vi "zmq_config_curve.vi"(4 "domain (none)":string, 5 "server public":string, 6 "error in":errorcluster, 7 "public in":string, 8 "secret in":string, 9 "socket in":refnum<class "Socket.lvclass">) -> (0 "error out":errorcluster, 1 "public out":string, 2 "secret out":string, 3 "socket out":refnum<class "Socket.lvclass">)   [LabVIEW 2025, in "ZeroMQ.lvlib" / "Socket.lvclass"]
doc: "Configures a socket for CURVE authentication. If the server (public) key is provided, then the socket is configured as a client, otherwise it is configured as a server.\n\nPublic and private keys can be manually specified, and are automatically generated if not provided.\n\nKeys are encoded in Z85 format.\n\nDomain <b>should</b> be specified for authentication purposes.\n\nDetailed API documentation: http://api.zeromq.org/master:zmq-curve"
uses:
  Socket.lvclass
  Socket.lvclass/Socket.ctl
  socket_options.ctl
  ZeroMQ.lvlib
panel:
  # "ØMQ"
  # "labview"
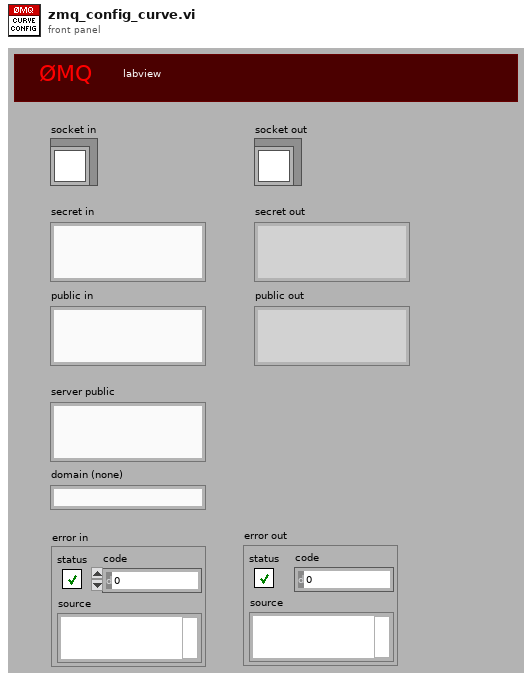
[diagram p1: front panel]
types:
  T1 = typedef "ZeroMQ.lvlib/socket_options.ctl" = enum8{"NONE", "ZMQ_HWM", "<2>", "ZMQ_SWAP", "ZMQ_AFFINITY", "ZMQ_ROUTING_ID", "ZMQ_SUBSCRIBE", "ZMQ_UNSUBSCRIBE", "ZMQ_RATE", "ZMQ_RECOVERY_IVL", "ZMQ_MCAST_LOOP", "ZMQ_SNDBUF", "ZMQ_RCVBUF", "ZMQ_RCVMORE", "ZMQ_FD", "ZMQ_EVENTS", "ZMQ_TYPE", "ZMQ_LINGER", "ZMQ_RECONNECT_IVL", "ZMQ_BACKLOG", "ZMQ_RECOVERY_IVL_MSEC", "ZMQ_RECONNECT_IVL_MAX", "ZMQ_MAXMSGSIZE", "ZMQ_SNDHWM", "ZMQ_RCVHWM", "ZMQ_MULTICAST_HOPS", "<26>", "ZMQ_RCVTIMEO", "ZMQ_SNDTIMEO", "<29>", "<30>", "ZMQ_IPV4ONLY", "ZMQ_LAST_ENDPOINT", "ZMQ_ROUTER_MANDATORY", "ZMQ_TCP_KEEPALIVE", "ZMQ_TCP_KEEPALIVE_CNT", "ZMQ_TCP_KEEPALIVE_IDLE", "ZMQ_TCP_KEEPALIVE_INTVL", "ZMQ_TCP_ACCEPT_FILTER", "ZMQ_IMMEDIATE", "ZMQ_XPUB_VERBOSE", "ZMQ_ROUTER_RAW", "ZMQ_IPV6", "ZMQ_MECHANISM", "ZMQ_PLAIN_SERVER", "ZMQ_PLAIN_USERNAME", "ZMQ_PLAIN_PASSWORD", "ZMQ_CURVE_SERVER", "ZMQ_CURVE_PUBLICKEY", "ZMQ_CURVE_SECRETKEY", "ZMQ_CURVE_SERVERKEY", "ZMQ_PROBE_ROUTER", "ZMQ_REQ_CORRELATE", "ZMQ_REQ_RELAXED", "ZMQ_CONFLATE", "ZMQ_ZAP_DOMAIN", "ZMQ_ROUTER_HANDOVER", "ZMQ_TOS", "ZMQ_IPC_FILTER_PID", "ZMQ_IPC_FILTER_UID", "ZMQ_IPC_FILTER_GID", "ZMQ_CONNECT_ROUTING_ID", "ZMQ_GSSAPI_SERVER", "ZMQ_GSSAPI_PRINCIPAL", "ZMQ_GSSAPI_SERVICE_PRINCIPAL", "ZMQ_GSSAPI_PLAINTEXT", "ZMQ_HANDSHAKE_IVL", "<67>", "ZMQ_SOCKS_PROXY", "ZMQ_XPUB_NODROP", "ZMQ_BLOCKY", "ZMQ_XPUB_MANUAL", "ZMQ_XPUB_WELCOME_MSG", "ZMQ_STREAM_NOTIFY", "ZMQ_INVERT_MATCHING", "ZMQ_HEARTBEAT_IVL", "ZMQ_HEARTBEAT_TTL", "ZMQ_HEARTBEAT_TIMEOUT", "ZMQ_XPUB_VERBOSER", "ZMQ_CONNECT_TIMEOUT", "ZMQ_TCP_MAXRT", "ZMQ_THREAD_SAFE", "<82>", "<83>", "ZMQ_MULTICAST_MAXTPDU", "ZMQ_VMCI_BUFFER_SIZE", "ZMQ_VMCI_BUFFER_MIN_SIZE", "ZMQ_VMCI_BUFFER_MAX_SIZE", "ZMQ_VMCI_CONNECT_TIMEOUT", "ZMQ_USE_FD", "ZMQ_GSSAPI_PRINCIPAL_NAMETYPE", "ZMQ_GSSAPI_SERVICE_PRINCIPAL_NAMETYPE", "ZMQ_BINDTODEVICE", "ZMQ_ZAP_ENFORCE_DOMAIN", "ZMQ_LOOPBACK_FASTPATH", "ZMQ_METADATA", "ZMQ_MULTICAST_LOOP", "ZMQ_ROUTER_NOTIFY"}
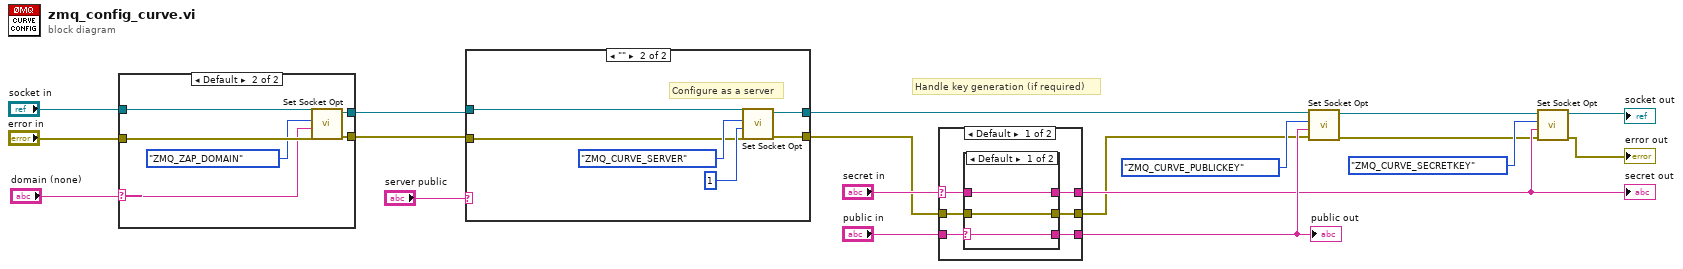
[diagram p0: block diagram]
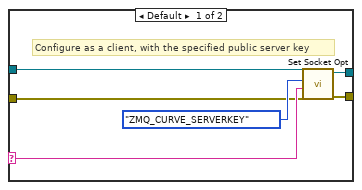
[diagram p3: hidden frame]
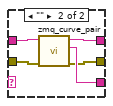
[diagram p4: hidden frame]
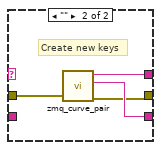
[diagram p5: hidden frame]
diagram:
  # "Handle key generation (if required)"
  n1 = case shown="Default" "domain (none)" {
    selector: "domain (none)" -> [_ w22]
    tunnel: "socket in" -> [w21 w27]
    tunnel: [w21 w26] -> w4
    tunnel: "error in" -> [w20 w25]
    tunnel: [w20 w24] -> w2
    frame "" {
    }
    frame Default {
      n2 = call "Set Socket Opt.vi"("error in"=w25, "value"=w22, "Socket option"=socket_options."ZMQ_ZAP_DOMAIN" ("option"), "socket in"=w27) -> ("error out"=w24:errorcluster, "socket out"=w26:refnum<class "Socket.lvclass">)  [unwired: 6 in]
    }
  }
  n3 = case shown="\"\"" "server public" {
    selector: "server public" -> [w32 _]
    tunnel: w4 -> [w28 w39]
    tunnel: w2 -> [w29 w36]
    tunnel: [w31 w35] -> w12
    tunnel: [w30 w34] -> w6
    frame Default {
      # "Configure as a client, with the specified public server key"
      n4 = call "Set Socket Opt.vi"("error in"=w29, "value"=w32, "Socket option"=socket_options."ZMQ_CURVE_SERVERKEY" ("option"), "socket in"=w28) -> ("error out"=w30:errorcluster, "socket out"=w31:refnum<class "Socket.lvclass">)  [unwired: 6 in]
    }
    frame "" {
      # "Configure as a server"
      n5 = call "Set Socket Opt.vi"("error in"=w36, "value"=1, "Socket option"=socket_options."ZMQ_CURVE_SERVER" ("option"), "socket in"=w39) -> ("error out"=w34:errorcluster, "socket out"=w35:refnum<class "Socket.lvclass">)  [unwired: 6 in]
    }
  }
  n6 = case shown="Default" "secret in" {
    selector: "secret in" -> [w44 _]
    tunnel: "public in" -> [w45 _]
    tunnel: [w43 w57] -> w13
    tunnel: [w42 w56] -> w14
    tunnel: w6 -> [w41 w55]
    tunnel: [w40 w54] -> w7
    frame Default {
      n7 = case shown="Default" w45 {
        selector: w45 -> [w48 _]
        tunnel: w44 -> [w47 w53]
        tunnel: [w47 w52] -> w43
        tunnel: [w48 w51] -> w42
        tunnel: w41 -> [w46 w50]
        tunnel: [w46 w49] -> w40
        frame Default {
        }
        frame "" {
          n8 = call "zmq_curve_pair.vi"("error in"=w50, "secret in"=w53) -> ("error out"=w49:errorcluster, "public out"=w51:string, "secret out"=w52:string)  [unwired: 7 in]
        }
      }
    }
    frame "" {
      # "Create new keys"
      n9 = call "zmq_curve_pair.vi"("error in"=w55) -> ("error out"=w54:errorcluster, "public out"=w56:string, "secret out"=w57:string)  [unwired: 8 in]
    }
  }
  "public out" <- w14
  "secret out" <- w13
  n10 = call "Set Socket Opt.vi"("error in"=w7, "value"=w14, "Socket option"=socket_options."ZMQ_CURVE_PUBLICKEY" ("option"), "socket in"=w12) -> ("error out"=w10:errorcluster, "socket out"=w11:refnum<class "Socket.lvclass">)  [unwired: 6 in]
  n11 = call "Set Socket Opt.vi"("error in"=w10, "value"=w13, "Socket option"=socket_options."ZMQ_CURVE_SECRETKEY" ("option"), "socket in"=w11) -> ("error out"=→"error out":errorcluster, "socket out"=→"socket out":refnum<class "Socket.lvclass">)  [unwired: 6 in]
